vi "SetParam.vi"(8 "error in (no error)":errorcluster caption="entrée d'erreur (pas d'erreur)", 10 "make_blobs":T1={"n_samples"=[100], "n_features"=2, "centers"=[], "cluster_std"=[], "centermin"=-10.0, "centermax"=10.0, "shuffle"=TRUE, "random_state"=-1, "Returns"="X"} {"random_state" min=-1; "n_features" min=1}, 11 "Blobs.lvclass":refnum<class "Blobs.lvclass">) -> (0 "error out":errorcluster caption="sortie d'erreur", 3 "Blobs.lvclass":refnum<class "Blobs.lvclass">)   [LabVIEW 2020, in "Blobs.lvclass"]
doc: "Set Parameters"
uses:
  Blobs.lvclass
  Blobs.lvclass/Blobs.ctl
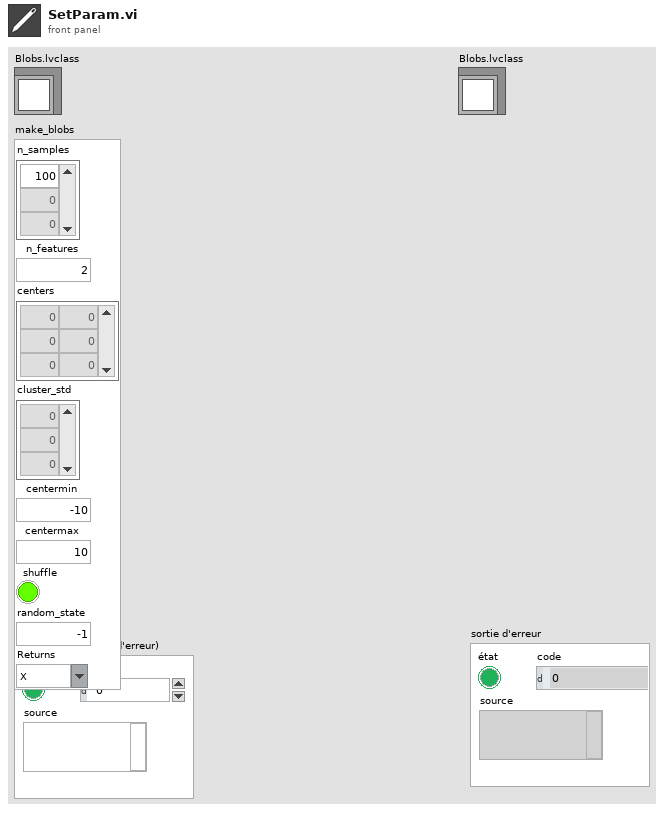
[diagram p1: front panel]
types:
  T1 = cluster{"n_samples":i32[], "n_features":u32, "centers":i32[][], "cluster_std":dbl[], "centermin":dbl, "centermax":dbl, "shuffle":bool, "random_state":i32, "Returns":string}
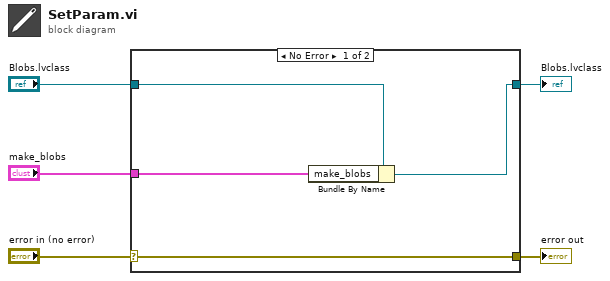
[diagram p0: block diagram]
diagram:
  n1 = case shown="No Error" "error in (no error)" {
    selector: "error in (no error)" -> [w9 w10]
    tunnel: [w9 w10] -> w4
    tunnel: [w7 w11] -> w2
    tunnel: "Blobs.lvclass" -> [w8 w11]
    tunnel: "make_blobs" -> [w6 _]
    frame No Error {
      n2 = Bundle By Name(cluster=w8, "make_blobs"=w6) -> (w7:refnum<class "Blobs.lvclass">)
    }
    frame Error {
    }
  }
  "error out" <- w4
  "Blobs.lvclass" <- w2
